vi "Get Scanner.vi"(8 "error in (no error)":errorcluster, 11 "Spectrometer Digikröm in":refnum<class "Spectrometer Digikröm.lvclass">) -> (0 "error out":errorcluster, 2 "Default Scanner out":refnum<class "Scanner.lvclass">)   [LabVIEW 2023, in "Spectrometer Digikröm.lvclass"]
doc: "(Dynamic) Returns the default Scanner object that scans over this Scannable. (Note that a Scannable may have multiple Scanners associated with it.) A Scanner is an analogue to an Iterator class in other languages."
uses:
  Scanners/Scanner/Scanner.lvclass
  C:/LabVIEW-programs/Scanners/Scanner/Scanner.lvclass
  Utility Classes/Scannable/Scannable.lvclass
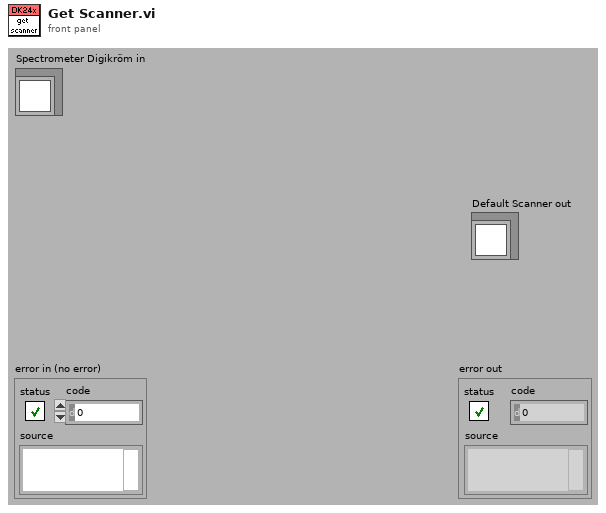
[diagram p1: front panel]
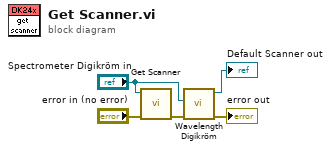
[diagram p0: block diagram]
diagram:
  n1 = call-parent "Get Scanner.vi"("error in (no error)"="error in (no error)", "Scannable in"="Spectrometer Digikröm in") -> ("error out"=w2:errorcluster)  [unwired: 9 out]
  n2 = call "Wavelength Digikröm.vi"("error in (no error)"=w2, "Spectrometer Digikröm.lvclass"="Spectrometer Digikröm in") -> ("error out"=→"error out":errorcluster, "Wavelength Digikröm out"=→"Default Scanner out":refnum<class "Wavelength Digikröm.lvclass">)  [unwired: 8 out]
